vi "Load Classes.vi"(8 "error in (no error)":errorcluster, 11 "Transceiver Loader in":refnum<class "Transceiver Loader.lvclass">) -> (0 "error out":errorcluster, 2 "Transceivers":refnum<class "Transceiver.lvclass">[](array[class]), 3 "Transceiver Loader out":refnum<class "Transceiver Loader.lvclass">)   [LabVIEW 2017, in "Data Sharing Framework Engine.lvlib" / "Transceiver Loader.lvclass"]
uses:
  Transceiver Loader.lvclass
  Transceiver/Transceiver.lvclass
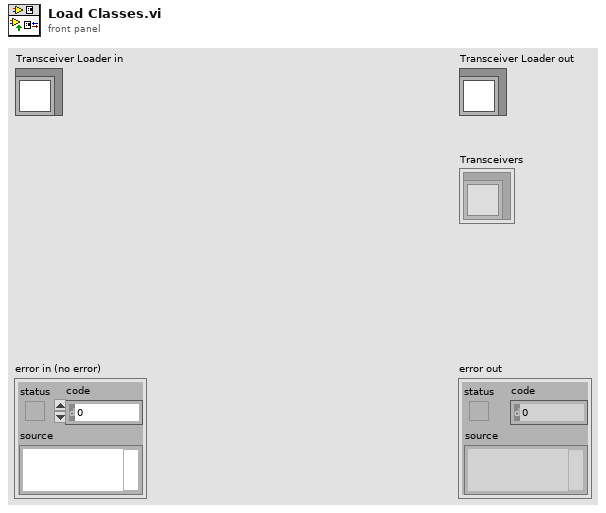
[diagram p1: front panel]
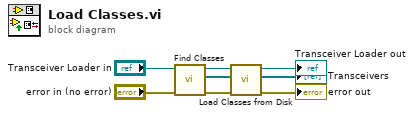
[diagram p0: block diagram]
diagram:
  n1 = call "Find Classes.vi"("error in (no error)"="error in (no error)", "Transceiver Loader in"="Transceiver Loader in") -> ("error out"=w6:errorcluster, "class paths"=w1:path[], "Transceiver Loader out"=w5:refnum<class "Transceiver Loader.lvclass">)  [unwired: 7 in]
  n2 = call "Load Classes from Disk.vi"("error in (no error)"=w6, "class paths"=w1, "Transceiver Loader in"=w5) -> ("error out"=→"error out":errorcluster, "Transceivers"=→"Transceivers":refnum<class "Transceiver.lvclass">[], "Transceiver Loader out"=→"Transceiver Loader out":refnum<class "Transceiver Loader.lvclass">)  [unwired: 6 in]
